vi "One_button_dialog.vi"(8 "error in (no error)":errorcluster, 11 "message":string) -> (0 "error out":errorcluster)   [LabVIEW 2019, in "SHARED VI'S.lvlib"]
uses:
  SHARED VI'S.lvlib
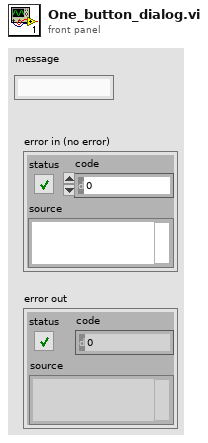
[diagram p1: front panel]
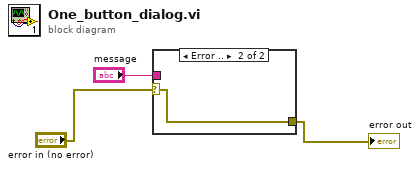
[diagram p0: block diagram]
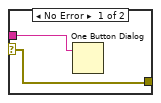
[diagram p2: hidden frame]
diagram:
  n1 = case shown="Error .." "error in (no error)" {
    selector: "error in (no error)" -> [w4 w6]
    tunnel: "message" -> [w5 _]
    tunnel: [w4 w6] -> w1
    frame No Error {
      n2 = One Button Dialog(message=w5) -> ()  [unwired: 1 in, 1 out]
    }
    frame Error {
    }
  }
  "error out" <- w1
